vi "Get Named Color.vi"(8 "error in (no error)":errorcluster, 11 "Named Colors":T1) -> (0 "error out":errorcluster, 3 "Color out":u32(colorbox))   [LabVIEW 2015, in "ColorSelector.lvclass"]
doc: "This VI looks up the color by name in a color lookup table. This are traditional names for these colors. The names are defined by the <b>Named Colors Enum.ctl</b>.\n<b> </b> <b> </b>\n©2017 Q Software Innovations, LLC (QSI)\nwritten by Quentin Alldredge\nproduced in LabVIEW 2015\n\nsupport@qsoftwareinnovations.com\nwww.qsoftwareinnovations.com\n\nAll rights reserved.\n\nRedistribution and use in source and binary forms, with or without modification, are permitted provided that the following conditions are met:\n\n * Redistributions of source code must retain the above copyright notice, this list of conditions and the following disclaimer.\n * Redistributions in binary form must reproduce the above copyright notice, this list of conditions and the following disclaimer in the documentation and/or other materials provided with the distribution.\n * Neither the name of Q Software Innovations, LLC. nor the names of its contributors may be used to endorse or promote products derived from this software without specific prior written permission.\n\nTHIS SOFTWARE IS PROVIDED BY THE COPYRIGHT HOLDERS AND CONTRIBUTORS \"AS IS\" AND ANY EXPRESS OR IMPLIED WARRANTIES, INCLUDING, BUT NOT LIMITED TO, THE IMPLIED WARRANTIES OF MERCHANTABILITY AND FITNESS FOR A PARTICULAR PURPOSE ARE DISCLAIMED. IN NO EVENT SHALL THE COPYRIGHT OWNER OR CONTRIBUTORS BE LIABLE FOR ANY DIRECT, INDIRECT, INCIDENTAL, SPECIAL, EXEMPLARY, OR CONSEQUENTIAL DAMAGES (INCLUDING, BUT NOT LIMITED TO, PROCUREMENT OF SUBSTITUTE GOODS OR SERVICES; LOSS OF USE, DATA, OR PROFITS; OR BUSINESS INTERRUPTION) HOWEVER CAUSED AND ON ANY THEORY OF LIABILITY, WHETHER IN CONTRACT, STRICT LIABILITY, OR TORT (INCLUDING NEGLIGENCE OR OTHERWISE) ARISING IN ANY WAY OUT OF THE USE OF THIS SOFTWARE, EVEN IF ADVISED OF THE POSSIBILITY OF SUCH DAMAGE."
uses:
  ColorSelector.lvclass
  Named Colors Enum.ctl
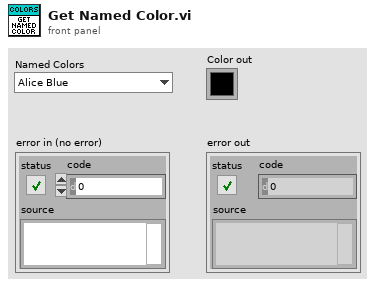
[diagram p1: front panel]
types:
  T1 = typedef "ColorSelector.lvclass/Named Colors Enum.ctl" = enum16{"Alice Blue", "Antique White", "Aqua Marine", "Azure", "Beige", "Bisque", "Black", "Blanched Almond", "Blue", "Blue Violet", "Brown", "Burly Wood", "Cadet Blue", "Chart Reuse", "Chocolate", "Coral", "Corn Flower Blue", "Corn Silk", "Crimson", "Cyan / Aqua", "Dark Blue", "Dark Cyan", "Dark Golden Rod", "Dark Gray / Dark Grey", "Dark Green", "Dark Khaki", "Dark Magenta", "Dark Olive Green", "Dark Orange", "Dark Orchid", "Dark Red", "Dark Salmon", "Dark Sea Green", "Dark Slate Blue", "Dark Slate Gray", "Dark Turquoise", "Dark Violet", "Deep Pink", "Deep Sky Blue", "Dim Gray / Dim Grey", "Dodger Blue", "Firebrick", "Floral White", "Forest Green", "Gainsboro", "Ghost White", "Gold", "Golden Rod", "Gray / Grey", "Green", "Green Yellow", "Honeydew", "Hot Pink", "Indian Red", "Indigo", "Ivory", "Khaki", "Lavender", "Lavender Blush", "Lawn Green", "Lemon Chiffon", "Light Blue", "Light Coral", "Light Cyan", "Light Golden Rod Yellow", "Light Gray / Light Grey", "Light Green", "Light Pink", "Light Salmon", "Light Sea Green", "Light Sky Blue", "Light Slate Gray", "Light Steel Blue", "Light Yellow", "Lime", "Lime Green", "Linen", "Magenta / Fuchsia", "Maroon", "Medium Aqua Marine", "Medium Blue", "Medium Orchid", "Medium Purple", "Medium Sea Green", "Medium Slate Blue", "Medium Spring Green", "Medium Turquoise", "Medium Violet Red", "Midnight Blue", "Mint Cream", "Misty Rose", "Moccasin", "Navajo White", "Navy", "Old Lace", "Olive", "Olive Drab", "Orange", "Orange Red", "Orchid", "Pale Golden Rod", "Pale Green", "Pale Turquoise", "Pale Violet Red", "Papaya Whip", "Peach Puff", "Peru", "Pink", "Plum", "Powder Blue", "Purple", "RYB Primary Blue", "RYB Primary Red", "RYB Primary Yellow", "RYB Secondary Green", "RYB Secondary Orange", "RYB Secondary Purple", "RYB Tertiary Amber", "RYB Tertiary Chartreuse", "RYB Tertiary Magenta", "RYB Tertiary Teal", "RYB Tertiary Vermillion", "RYB Tertiary Violet", "Red", "Rosy Brown", "Royal Blue", "Saddle Brown", "Salmon", "Sandy Brown", "Sea Green", "Sea Shell", "Sienna", "Silver", "Sky Blue", "Slate Blue", "Slate Gray", "Snow", "Spring Green", "Steel Blue", "Tan", "Teal", "Thistle", "Tomato", "Turquoise", "Violet", "Wheat", "White", "White Smoke", "Yellow", "Yellow Green"}
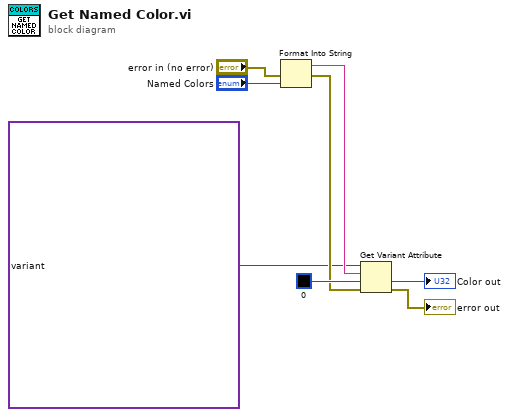
[diagram p0: block diagram]
diagram:
  n1 = Format Into String(error in="error in (no error)", "Named Colors") -> (resulting string=w7:string, error out=w4:errorcluster)  [unwired: 2 in]
  n2 = Get Variant Attribute(Variant=variant("Alice Blue"=variant(u32 15792383), "Antique White"=variant(u32 16444375), "Aqua Marine"=variant(u32 8388564), "Azure"=variant(u32 15794175), "Beige"=variant(u32 16119260), "Bisque"=variant(u32 16770244), "Black"=variant(u32 0), "Blanched Almond"=variant(u32 16772045), "Blue"=variant(u32 255), "Blue Violet"=variant(u32 9055202), "Brown"=variant(u32 10824234), "Burly Wood"=variant(u32 14596231), "Cadet Blue"=variant(u32 6266528), "Chart Reuse"=variant(u32 8388352), "Chocolate"=variant(u32 13789470), "Coral"=variant(u32 16744272), "Corn Flower Blue"=variant(u32 6591981), "Corn Silk"=variant(u32 16775388), "Crimson"=variant(u32 14423100), "Cyan / Aqua"=variant(u32 65535), "Dark Blue"=variant(u32 139), "Dark Cyan"=variant(u32 35723), "Dark Golden Rod"=variant(u32 12092939), "Dark Gray / Dark Grey"=variant(u32 11119017), "Dark Green"=variant(u32 25600), "Dark Khaki"=variant(u32 12433259), "Dark Magenta"=variant(u32 9109643), "Dark Olive Green"=variant(u32 5597999), "Dark Orange"=variant(u32 16747520), "Dark Orchid"=variant(u32 10040012), "Dark Red"=variant(u32 9109504), "Dark Salmon"=variant(u32 15308410), "Dark Sea Green"=variant(u32 9419919), "Dark Slate Blue"=variant(u32 4734347), "Dark Slate Gray"=variant(u32 3100495), "Dark Turquoise"=variant(u32 52945), "Dark Violet"=variant(u32 9699539), "Deep Pink"=variant(u32 16716947), "Deep Sky Blue"=variant(u32 49151), "Dim Gray / Dim Grey"=variant(u32 6908265), "Dodger Blue"=variant(u32 2003199), "Firebrick"=variant(u32 11674146), "Floral White"=variant(u32 16775920), "Forest Green"=variant(u32 2263842), "Gainsboro"=variant(u32 14474460), "Ghost White"=variant(u32 16316671), "Gold"=variant(u32 16766720), "Golden Rod"=variant(u32 14329120), "Gray / Grey"=variant(u32 8421504), "Green"=variant(u32 32768), "Green Yellow"=variant(u32 11403055), "Honeydew"=variant(u32 15794160), "Hot Pink"=variant(u32 16738740), "Indian Red"=variant(u32 13458524), "Indigo"=variant(u32 4915330), "Ivory"=variant(u32 16777200), "Khaki"=variant(u32 15787660), "Lavender"=variant(u32 15132410), "Lavender Blush"=variant(u32 16773365), "Lawn Green"=variant(u32 8190976), "Lemon Chiffon"=variant(u32 16775885), "Light Blue"=variant(u32 11393254), "Light Coral"=variant(u32 15761536), "Light Cyan"=variant(u32 14745599), "Light Golden Rod Yellow"=variant(u32 16448210), "Light Gray / Light Grey"=variant(u32 13882323), "Light Green"=variant(u32 9498256), "Light Pink"=variant(u32 16758465), "Light Salmon"=variant(u32 16752762), "Light Sea Green"=variant(u32 2142890), "Light Sky Blue"=variant(u32 8900346), "Light Slate Gray"=variant(u32 7833753), "Light Steel Blue"=variant(u32 11584734), "Light Yellow"=variant(u32 16777184), "Lime"=variant(u32 65280), "Lime Green"=variant(u32 3329330), "Linen"=variant(u32 16445670), "Magenta / Fuchsia"=variant(u32 16711935), "Maroon"=variant(u32 8388608), "Medium Aqua Marine"=variant(u32 6737322), "Medium Blue"=variant(u32 205), "Medium Orchid"=variant(u32 12211667), "Medium Purple"=variant(u32 9662683), "Medium Sea Green"=variant(u32 3978097), "Medium Slate Blue"=variant(u32 8087790), "Medium Spring Green"=variant(u32 64154), "Medium Turquoise"=variant(u32 4772300), "Medium Violet Red"=variant(u32 13047173), "Midnight Blue"=variant(u32 1644912), "Mint Cream"=variant(u32 16121850), "Misty Rose"=variant(u32 16770273), "Moccasin"=variant(u32 16770229), "Navajo White"=variant(u32 16768685), "Navy"=variant(u32 128), "Old Lace"=variant(u32 16643558), "Olive"=variant(u32 8421376), "Olive Drab"=variant(u32 7048739), "Orange"=variant(u32 16753920), "Orange Red"=variant(u32 16729344), "Orchid"=variant(u32 14315734), "Pale Golden Rod"=variant(u32 15657130), "Pale Green"=variant(u32 10025880), "Pale Turquoise"=variant(u32 11529966), "Pale Violet Red"=variant(u32 14381203), "Papaya Whip"=variant(u32 16773077), "Peach Puff"=variant(u32 16767673), "Peru"=variant(u32 13468991), "Pink"=variant(u32 16761035), "Plum"=variant(u32 14524637), "Powder Blue"=variant(u32 11591910), "Purple"=variant(u32 8388736), "RYB Primary Blue"=variant(u32 2777241), "RYB Primary Red"=variant(u32 16711680), "RYB Primary Yellow"=variant(u32 16776960), "RYB Secondary Green"=variant(u32 43571), "RYB Secondary Orange"=variant(u32 16744448), "RYB Secondary Purple"=variant(u32 8388736), "RYB Tertiary Amber"=variant(u32 16760576), "RYB Tertiary Chartreuse"=variant(u32 8442906), "RYB Tertiary Magenta"=variant(u32 12517441), "RYB Tertiary Teal"=variant(u32 1410150), "RYB Tertiary Vermillion"=variant(u32 16733001), "RYB Tertiary Violet"=variant(u32 5582989), "Red"=variant(u32 16711680), "Rosy Brown"=variant(u32 12357519), "Royal Blue"=variant(u32 4286945), "Saddle Brown"=variant(u32 9127187), "Salmon"=variant(u32 16416882), "Sandy Brown"=variant(u32 16032864), "Sea Green"=variant(u32 3050327), "Sea Shell"=variant(u32 16774638), "Sienna"=variant(u32 10506797), "Silver"=variant(u32 12632256), "Sky Blue"=variant(u32 8900331), "Slate Blue"=variant(u32 6970061), "Slate Gray"=variant(u32 7372944), "Snow"=variant(u32 16775930), "Spring Green"=variant(u32 65407), "Steel Blue"=variant(u32 4620980), "Tan"=variant(u32 13808780), "Teal"=variant(u32 32896), "Thistle"=variant(u32 14204888), "Tomato"=variant(u32 16737095), "Turquoise"=variant(u32 4251856), "Violet"=variant(u32 15631086), "Wheat"=variant(u32 16113331), "White"=variant(u32 16777215), "White Smoke"=variant(u32 16119285), "Yellow"=variant(u32 16776960), "Yellow Green"=variant(u32 10145074)), name=w7, default value (empty Variant)=u32 0, error in=w4) -> (value=→"Color out":u32, error out=→"error out":errorcluster)  [unwired: 2 out]
